vi "MPXsetOnOff.vi"(2 "Refresh":bool, 3 "Signal On":bool, 4 "Comport in":refnum<visa-resource-name>="COM5") -> (0 "read buffer":string="A198,0\r\nAmplitude changed\r\n\r\nWavetype: Sine\r\nFrequence: 0125 Hz\r\nAmplitude: 198,0 V\r\nSignal off\r\n\r\nempc>:\n", 1 "Comport out":refnum<visa-resource-name>="COM5")   [LabVIEW 2015]
panel:
  out "Signal on bkp":bool
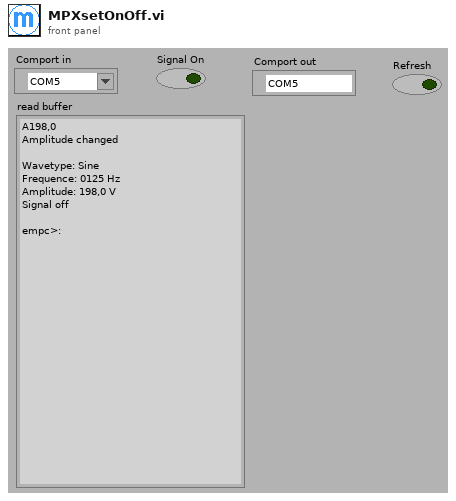
[diagram p1: front panel]
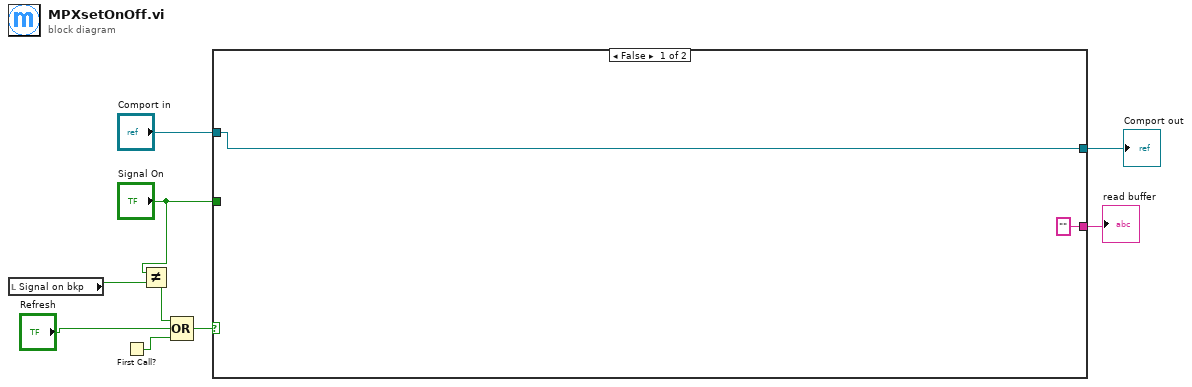
[diagram p0: block diagram]
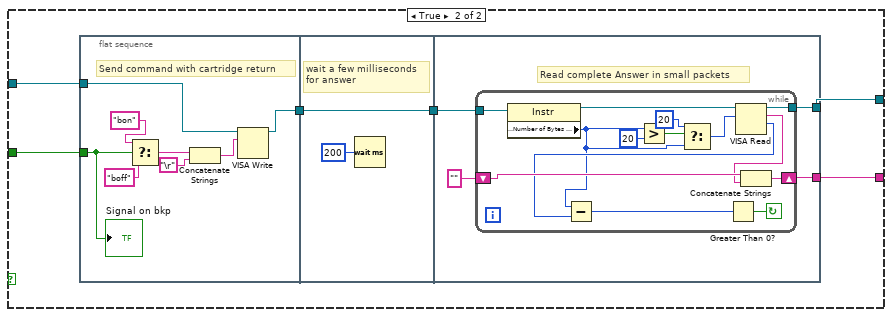
[diagram p2: hidden frame]
diagram:
  n1 = local read "Signal on bkp"() -> (w3:bool)
  n2 = First Call?() -> (First Call?: T/F=w4:bool)
  n3 = Not Equal?(x="Signal On", y=w3) -> (x != y?=w5:bool)
  n4 = Compound Arithmetic op=OR(w5, "Refresh", w4) -> (w7:bool)
  n5 = case shown="False" w7 {
    tunnel: "Comport in" -> [w11 w15]
    tunnel: "Signal On" -> [_ w14]
    tunnel: [w11 w13] -> w8
    tunnel: ["" w12] -> w1
    frame False {
    }
    frame True {
      n6 = flat-sequence {
        tunnel: w15 -> [w20]
        tunnel: [w19] -> w17
        tunnel: w14 -> [w18]
        tunnel: w17 -> [w26]
        tunnel: [w26] -> w16
        tunnel: w16 -> [w31]
        tunnel: [w29] -> w12
        tunnel: [w28] -> w13
        frame #0 {
          # "Send command with cartridge return"
          n7 = Select(t="bon", s=w18, f="boff") -> (s? t:f=w23:string)
          n8 = Concatenate Strings(w23, "\r") -> (w25:string)
          n9 = VISA Write(VISA resource name=w20, write buffer=w25) -> (VISA resource name out=w19:refnum<visa-resource-name>)  [unwired: 1 in, 2 out]
          "Signal on bkp" <- w18
        }
        frame #1 {
          # "wait a few milliseconds\nfor answer"
          n10 = Wait (ms)(milliseconds to wait=u32 200) -> ()  [unwired: 1 out]
        }
        frame #2 {
          # "Read complete Answer in small packets"
          n11 = while {
            shift-right: [w43] -> w29
            shift-left: "" -> [w44]
            tunnel: w31 -> [w38]
            tunnel: [w32] -> w28
            stop <- w39 continue-if-true
            n12 = property class="Instr"(reference=w38) -> (reference out=w45:refnum<visa-resource-name>, "Serial Settings:Number of Bytes at Serial Port"=w37:u32)  [unwired: 1 in, 1 out]
            n13 = Greater?(x=w37, y=u32 20) -> (0:w35:bool)
            n14 = Select(t=u32 20, s=w35, f=w37) -> (s? t:f=w36:u32)
            n15 = VISA Read(VISA resource name=w45, byte count=w36) -> (VISA resource name out=w32:refnum<visa-resource-name>, read buffer=w42:string, return count=w40:u32)  [unwired: 1 in, 1 out]
            n16 = Subtract(x=w37, y=w40) -> (x-y=w41:u32)
            n17 = Greater Than 0?(x=w41) -> (x > 0?=w39:bool)
            n18 = Concatenate Strings(w44, w42) -> (w43:string)
          }
        }
      }
    }
  }
  "Comport out" <- w8
  "read buffer" <- w1
